vi "Periodic Tasks.vi"(8 "error in":errorcluster) -> ()   [LabVIEW 2016]
doc: "This VI runs in parallel to other tasks. It can contain as many user-defined periodic loops as you need. These can carry out PID or other sorts of timed response."
uses:
  <vilib>/Rock Robotics/WPI/Solenoid/WPI_SolenoidValue.ctl
  <vilib>/Rock Robotics/Network Tables/NT Read Number.vi
  <vilib>/Rock Robotics/WPI/Utilities/WPI_GetSetVariantRefNum.vi
  <vilib>/Rock Robotics/WPI/Solenoid/WPI_SolenoidSetEnum.vi
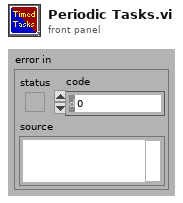
[diagram p1: front panel]
types:
  T1 = typedef "WPI_JoystickDevRef.ctl" = cluster{"Device":T2}
  T2 = typedef "WPI_JoystickDeviceEnum.ctl" = enum16{"USB 0", "USB 1", "USB 2", "USB 3", "USB 4", "USB 5"}
  T3 = typedef "WPI_MotorControlDeviceRef.ctl" = cluster{"DeviceStatus":errorcluster, "Type":T4, "PWM":cluster{"PWM Channel":T5, "DeadBand":T6}, "CAN":cluster{"Device Number":u8, "SetOutput VI Ref":variant, "GetOutput VI Ref":variant, "Enable VI Ref":variant, "Disable VI Ref":variant, "Data":variant}, "Invert":bool}
  T4 = typedef "WPI_MotorControlType.ctl" = enum16{"PWM", "CAN"}
  T5 = typedef "FPGA_DIOPWMChannel.ctl" = enum8{"PWM 0", "PWM 1", "PWM 2", "PWM 3", "PWM 4", "PWM 5", "PWM 6", "PWM 7", "PWM 8", "PWM 9", "PWM MXP 0", "PWM MXP 1", "PWM MXP 2", "PWM MXP 3", "PWM MXP 4", "PWM MXP 5", "PWM MXP 6", "PWM MXP 7", "PWM MXP 8", "PWM MXP 9", "Invalid"}
  T6 = typedef "WPI_PWMDeadband.ctl" = cluster{"Name":string, "maxPositivePwm":i32, "minPositivePwm":i32, "centerPwm":i32, "maxNegativePwm":i32, "minNegativePwm":i32, "angularRange":u16}
  T7 = typedef "WPI_SolenoidDevRef.ctl" = cluster{"DevStatus":errorcluster, "Pneumatics Control Module":u8, "Forward Solenoid Channel":T8, "Reverse Solenoid Channel":T8}
  T8 = typedef "WPI_SolenoidChannel.ctl" = enum8{"Solenoid 0", "Solenoid 1", "Solenoid 2", "Solenoid 3", "Solenoid 4", "Solenoid 5", "Solenoid 6", "Solenoid 7", "Invalid"}
  T9 = typedef "WPI_SwitchDevRef.ctl" = cluster{"DevStatus":errorcluster, "DIO Channel":T10, "CntIndex":T11, "Normally Closed":bool}
  T10 = typedef "FPGA_DIOChannel.ctl" = enum8{"DIO 0", "DIO 1", "DIO 2", "DIO 3", "DIO 4", "DIO 5", "DIO 6", "DIO 7", "DIO 8", "DIO 9", "DIO MXP 0", "DIO MXP 1", "DIO MXP 2", "DIO MXP 3", "DIO MXP 4", "DIO MXP 5", "DIO MXP 6", "DIO MXP 7", "DIO MXP 8", "DIO MXP 9", "DIO MXP 10", "DIO MXP 11", "DIO MXP 12", "DIO MXP 13", "DIO MXP 14", "DIO MXP 15", "SPI Port CS1", "SPI Port CS2", "SPI Port CS3", "SPI Port MISO", "SPI Port MOSI", "Invalid"}
  T11 = typedef "FPGA_CounterCtrSystemIndex.ctl" = enum8{"Ctr 0", "Ctr 1", "Ctr 2", "Ctr 3", "Ctr 4", "Ctr 5", "Ctr 6", "Ctr 7", "Invalid"}
  T12 = typedef "WPI_SolenoidValue.ctl" = enum16{"Off", "On", "Forward", "Reverse"}
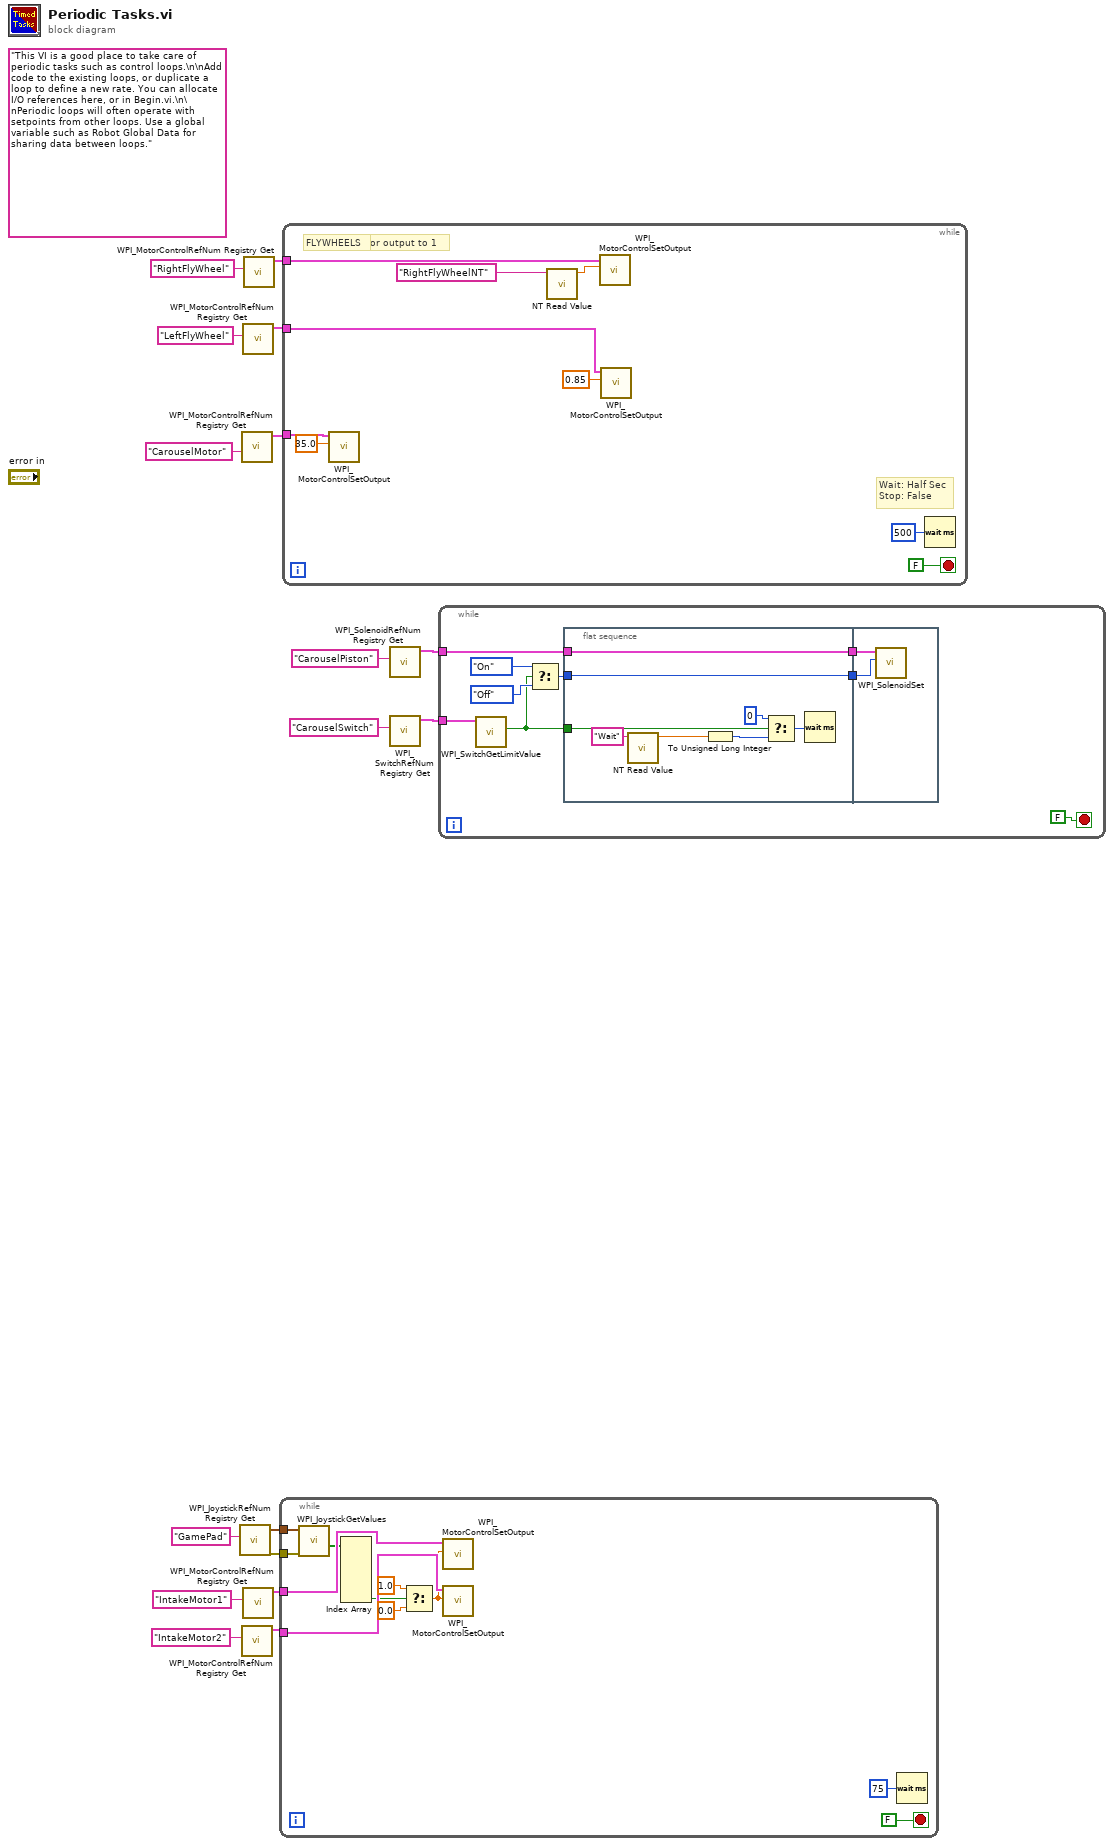
[diagram p0: block diagram]
diagram:
  (unwired) "This VI is a good place to take care of periodic tasks such as control loops.\n\nAdd code to the existing loops, or duplicate a loop to define a new rate. You can allocate I/O references here, or in Begin.vi.\n\nPeriodic loops will often operate with setpoints from other loops. Use a global variable such as Robot Global Data for sharing data between loops."
  n1 = call <vilib>:"WPI_JoystickRefNum Registry Get.vi"("refnum name"="GamePad") -> ("error out"=w3:errorcluster, "JoystickDevRef"=w2:T1)  [unwired: 9 in]
  n2 = call <vilib>:"WPI_MotorControlRefNum Registry Get.vi"("refnum name"="CarouselMotor") -> ("MotorControlDevRef"=w15:T3)  [unwired: 9 in, 1 out]
  n3 = call <vilib>:"WPI_MotorControlRefNum Registry Get.vi"("refnum name"="IntakeMotor2") -> ("MotorControlDevRef"=w5:T3)  [unwired: 9 in, 1 out]
  n4 = call <vilib>:"WPI_MotorControlRefNum Registry Get.vi"("refnum name"="LeftFlyWheel") -> ("MotorControlDevRef"=w16:T3)  [unwired: 9 in, 1 out]
  n5 = call <vilib>:"WPI_MotorControlRefNum Registry Get.vi"("refnum name"="IntakeMotor1") -> ("MotorControlDevRef"=w4:T3)  [unwired: 9 in, 1 out]
  n6 = call <vilib>:"WPI_MotorControlRefNum Registry Get.vi"("refnum name"="RightFlyWheel") -> ("MotorControlDevRef"=w17:T3)  [unwired: 9 in, 1 out]
  n7 = while {
    tunnel: w5 -> [w28]
    tunnel: w4 -> [w27]
    tunnel: w3 -> [w26]
    tunnel: w2 -> [w25]
    stop <- FALSE stop-if-true
    n8 = call <vilib>:"WPI_JoystickGetValues.vi"("error in (no error)"=w26, "JoystickDevRef"=w25) -> ("Buttons"=w24:bool[])  [unwired: 5 in, 4 out]
    n9 = Index Array(array=w24) -> (element #6=w23:bool)  [unwired: 6 in, 5 out]
    n10 = Select(t=1.0, s=w23, f=0.0) -> (s? t:f=w20:dbl)
    n11 = call <vilib>:"WPI_MotorControlSetOutput.vi"("Output"=w20, "MotorControlDevRef"=w27) -> ()  [unwired: 7 in, 3 out]
    n12 = call <vilib>:"WPI_MotorControlSetOutput.vi"("Output"=w20, "MotorControlDevRef"=w28) -> ()  [unwired: 7 in, 3 out]
    n13 = Wait (ms)(milliseconds to wait=u32 75) -> ()  [unwired: 1 out]
  }
  n14 = while {
    tunnel: w16 -> [w36]
    tunnel: w17 -> [w35]
    tunnel: w15 -> [w31]
    stop <- FALSE stop-if-true
    # "FLYWHEELS"
    # "Wait: Half Sec\nStop: False"
    # "Set right motor output to 1"
    n15 = call <vilib>:"WPI_MotorControlSetOutput.vi"("Output"=35.0, "MotorControlDevRef"=w31) -> ()  [unwired: 7 in, 3 out]
    n16 = call-poly <vilib>:"NT Read Value.vi"("Name"="RightFlyWheelNT") -> ("Numeric"=w32:dbl)  [unwired: 9 in, 1 out]
    n17 = call <vilib>:"WPI_MotorControlSetOutput.vi"("Output"=w32, "MotorControlDevRef"=w35) -> ()  [unwired: 7 in, 3 out]
    n18 = call <vilib>:"WPI_MotorControlSetOutput.vi"("Output"=0.85, "MotorControlDevRef"=w36) -> ()  [unwired: 7 in, 3 out]
    n19 = Wait (ms)(milliseconds to wait=u32 500) -> ()  [unwired: 1 out]
  }
  n20 = call <vilib>:"WPI_SolenoidRefNum Registry Get.vi"("refnum name"="CarouselPiston") -> ("SolenoidDevRef"=w10:T7)  [unwired: 9 in, 1 out]
  n21 = call <vilib>:"WPI_SwitchRefNum Registry Get.vi"("refnum name"="CarouselSwitch") -> ("SwitchDevRef"=w9:T9)  [unwired: 9 in, 1 out]
  n22 = while {
    tunnel: w9 -> [w45]
    tunnel: w10 -> [w44]
    stop <- FALSE stop-if-true
    n23 = call <vilib>:"WPI_SwitchGetLimitValue.vi"("SwitchDevRef"=w45) -> ("Switch Pressed"=w38:bool)  [unwired: 8 in, 2 out]
    n24 = Select(t=WPI_SolenoidValue."On" ("Value"), s=w38, f=WPI_SolenoidValue."Off" ("Value")) -> (s? t:f=w40:T12)
    n25 = flat-sequence {
      tunnel: w44 -> [w54]
      tunnel: [w54] -> w43
      tunnel: w40 -> [w53]
      tunnel: [w53] -> w39
      tunnel: w38 -> [w51]
      tunnel: w43 -> [w56]
      tunnel: w39 -> [w55]
      frame #0 {
        n26 = call-poly <vilib>:"NT Read Value.vi"("Name"="Wait") -> ("Numeric"=w48:dbl)  [unwired: 9 in, 1 out]
        n27 = To Unsigned Long Integer(number=w48) -> (unsigned 32bit integer=w49:u32)
        n28 = Select(t=u32 0, s=w51, f=w49) -> (s? t:f=w52:u32)
        n29 = Wait (ms)(milliseconds to wait=w52) -> ()  [unwired: 1 out]
      }
      frame #1 {
        n30 = call-poly <vilib>:"WPI_SolenoidSet.vi"("Value"=w55, "SolenoidDevRef"=w56) -> ()  [unwired: 8 in, 2 out]
      }
    }
  }
